vi "Data_Framing.vi"(10 "CAN_MSGs":T1={"Scaling Factor"=1, "Physical value"=0.0, "CAN_Frames"={"CAN_ID"=0, "MSGTYPE"=128, "Payload"=[], "Length"=0}, "Offset value"=0.0, "Framing datas"=[], "CAN_Frame Enable"=FALSE, "Add Signal"=FALSE, "Delete Signal"=FALSE, "Signal Values"=[], "Time(ms)"=0.0, "Repetition"=FALSE, "Delay"=FALSE, "Delay time"=0.0} {"CAN_Frames"."Payload" format="%.0x"; "CAN_Frames"."MSGTYPE" items=["STATUS"=128, "EXTENDED"=2, "RTR"=1, "DATA MSG"=0]; "CAN_Frames"."CAN_ID" format="%.0x"}) -> (1 "CAN_data frame":u8[](array[numeric]) format="%.0x", 2 "CAN_bit frame":bool[][](array[boolean]))   [LabVIEW 2024, in "PCANusb_DTU.lvlib"]
uses:
  PCANusb_DTU.lvlib
  CAN_MSGs.ctl
  CAN_Frames_ctrl.ctl
  Framing datas.ctl
panel:
  out "output array":bool[](array[boolean])
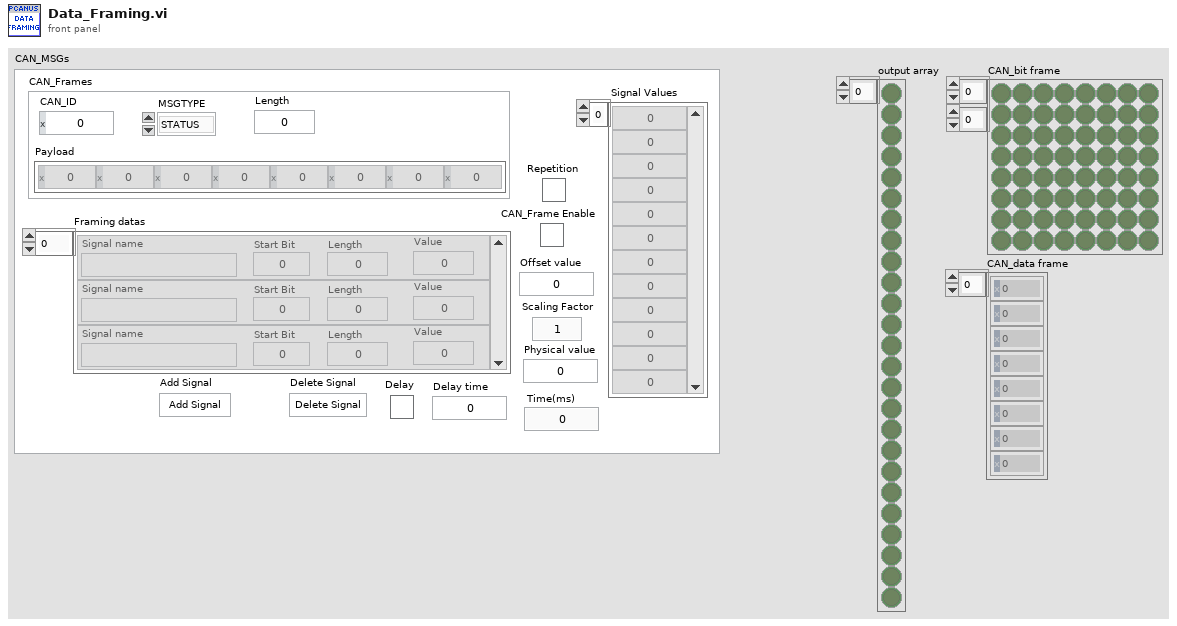
[diagram p1: front panel]
types:
  T1 = typedef "PCANusb_DTU.lvlib/CAN_MSGs.ctl" = cluster{"Scaling Factor":u16, "Physical value":dbl, "CAN_Frames":T2, "Offset value":dbl, "Framing datas":T3[], "CAN_Frame Enable":bool, "Add Signal":bool, "Delete Signal":bool, "Signal Values":dbl[], "Time(ms)":dbl, "Repetition":bool, "Delay":bool, "Delay time":dbl}
  T2 = typedef "PCANusb_DTU.lvlib/CAN_Frames_ctrl.ctl" = cluster{"CAN_ID":u32, "MSGTYPE":u8, "Payload":u8[], "Length":u8}
  T3 = typedef "PCANusb_DTU.lvlib/Framing datas.ctl" = cluster{"Signal name":string, "Start Bit":u8, "Length":u8, "Value":u16}
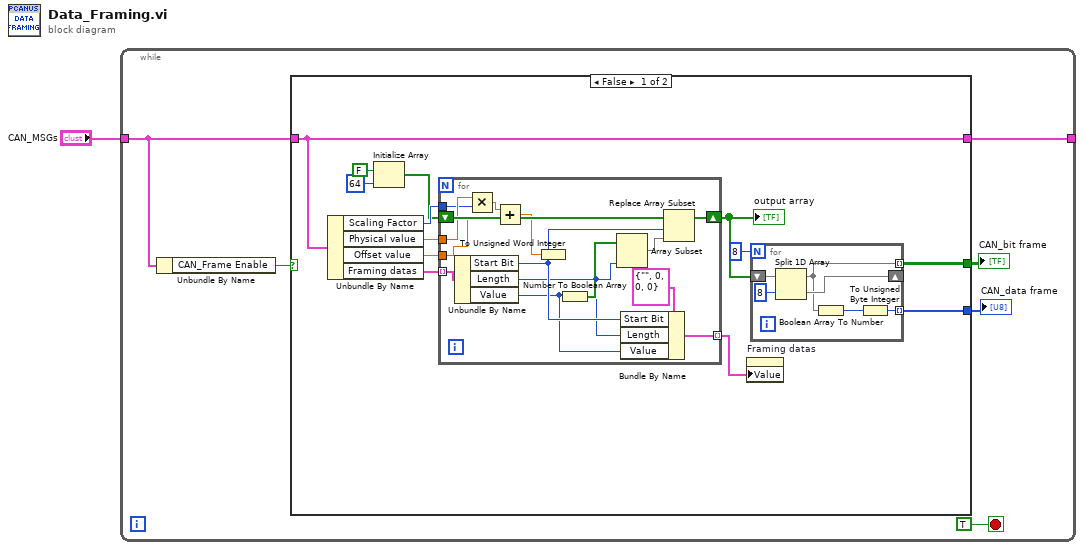
[diagram p0: block diagram]
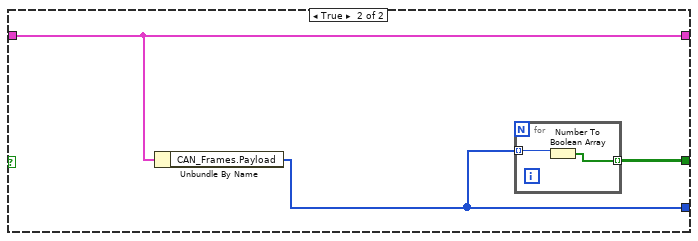
[diagram p2: hidden frame]
diagram:
  n1 = while {
    tunnel: "CAN_MSGs" -> [w5]
    tunnel: [w7] -> _
    stop <- TRUE stop-if-true
    n2 = Unbundle By Name(w5) -> ("CAN_Frame Enable"=w6:bool)
    n3 = case shown="False" w6 {
      tunnel: w5 -> [w20 w44]
      tunnel: [w20 w44] -> w7
      tunnel: [w9 w43] -> w3
      tunnel: [w8 w42] -> w2
      frame False {
        n4 = Unbundle By Name(w20) -> ("Scaling Factor"=w16:u16, "Physical value"=w18:dbl, "Offset value"=w17:dbl, "Framing datas"=w19:T3[])
        n5 = Initialize Array(FALSE, 64 ("dimension size")) -> (w13:bool[])
        n6 = for {
          tunnel: w19 -> [w41] mode=indexing
          tunnel: w18 -> [w32]
          tunnel: w17 -> [w29]
          tunnel: w16 -> [w31]
          shift-right: [w37] -> w12
          shift-left: w13 -> [w38]
          tunnel: [w33] -> w10 mode=indexing
          n7 = Unbundle By Name(w41) -> ("Start Bit"=w35:u8, "Length"=w34:u8, "Value"=w27:u16)
          n8 = Multiply(x=w32, y=w31) -> (x*y=w30:dbl)
          n9 = Add(x=w30, y=w29) -> (x+y=w28:dbl)
          n10 = To Unsigned Word Integer(number=w28) -> ()  [unwired: 1 out]
          n11 = Number To Boolean Array(number=w27) -> (Boolean array=w40:bool[])
          n12 = Array Subset(array=w40, length=w34) -> (w39:bool[])  [unwired: 1 in]
          n13 = Bundle By Name(cluster=T3 {"Signal name"="", "Start Bit"=0, "Length"=0, "Value"=0} ("Framing datas"), "Start Bit"=w35, "Length"=w34, "Value"=w27) -> (w33:T3)
          n14 = Replace Array Subset(array=w38, new element=w39, index=w35) -> (w37:bool[])
        }
        "output array" <- w12
        n15 = property on="Framing datas" class="Arr (strict)"("Value"=w10) -> ()  [unwired: 2 in, 2 out]
        n16 = for {
          N: 8 -> [_]
          shift-right: [w24] -> _
          shift-left: w12 -> [w26]
          tunnel: [w23] -> w8 mode=indexing
          tunnel: [w21] -> w9 mode=indexing
          n17 = Split 1D Array(array=w26, index=8) -> (first subarray=w23:bool[], second subarray=w24:bool[])
          n18 = Boolean Array To Number(Boolean array=w23) -> (number=w22:u32)
          n19 = To Unsigned Byte Integer(number=w22) -> (unsigned 8bit integer=w21:u8)
        }
      }
      frame True {
        n20 = Unbundle By Name(w44) -> ("CAN_Frames.Payload"=w43:u8[])
        n21 = for {
          tunnel: w43 -> [w46] mode=indexing
          tunnel: [w45] -> w42 mode=indexing
          n22 = Number To Boolean Array(number=w46) -> (Boolean array=w45:bool[])
        }
      }
    }
    "CAN_data frame" <- w3
    "CAN_bit frame" <- w2
  }
